vi "WaterValve.vi"(9 "Max pulses":u32=1, 11 "STOP":bool) -> (1 "Error":bool, 3 "Number pulses":u32)   [LabVIEW 2021]
uses:
  <vilib>/DAQmx/write.llb/DAQmx Write (Digital Bool 1Line 1Point).vi
  GlobalSTATE.vi
  <vilib>/DAQmx/create/channels.llb/DAQmx Create Channel (DO-Digital Output).vi
  Global_BeamBreaks.vi
  <vilib>/DAQmx/miscellaneous.llb/DAQmx Fill In Error Info.vi
panel:
  in  "Active":bool=TRUE
  in  "Min IPI":u32=500
  in  "Open time":u32=50
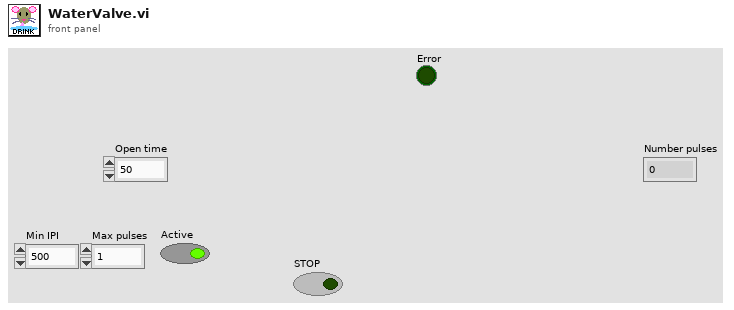
[diagram p1: front panel]
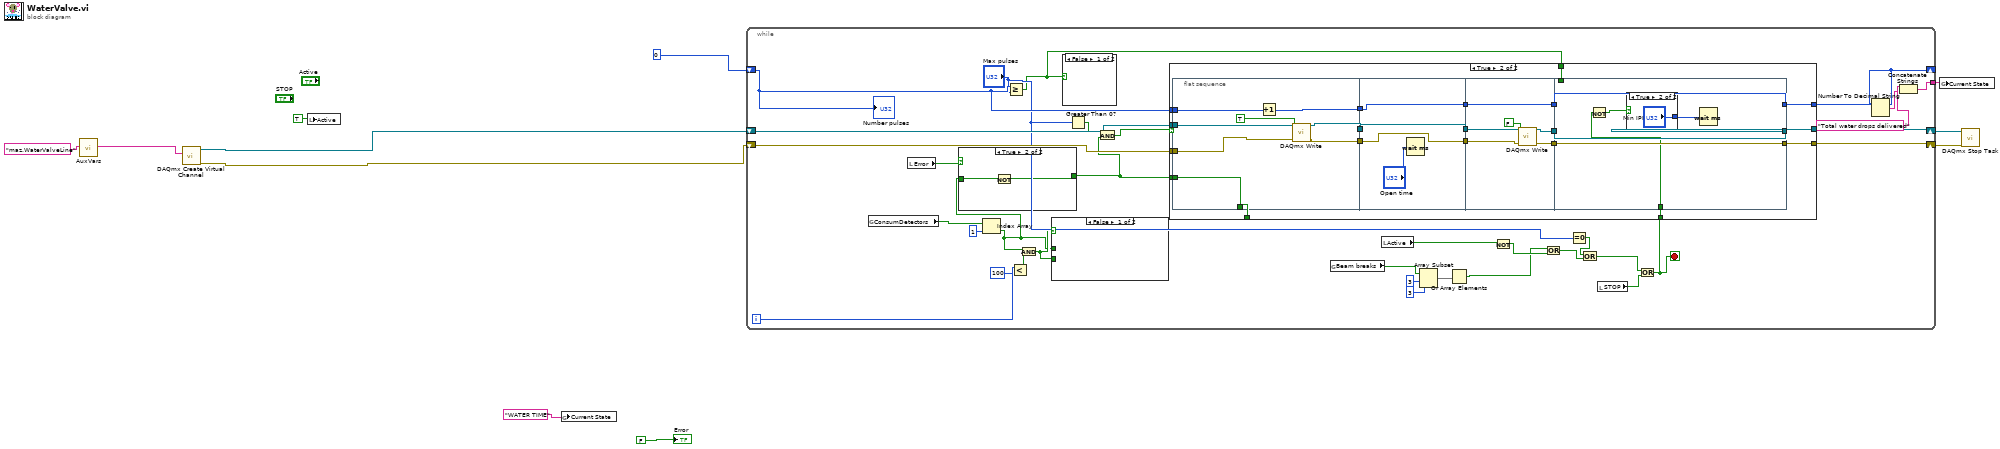
[diagram p0: block diagram]
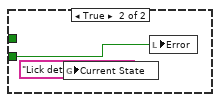
[diagram p3: hidden frame]
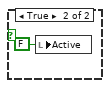
[diagram p4: hidden frame]
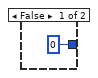
[diagram p6: hidden frame]
diagram:
  n1 = call "AuxVars.vi"("key"="maz.WaterValveLine") -> ("value"=w7:string)  [unwired: 9 in, 1 out]
  n2 = call-poly <vilib>:"DAQmx Create Virtual Channel.vi"("lines"=w7) -> ("task out"=w9:refnum<k21>, "error out"=w8:errorcluster)  [unwired: 13 in]
  n3 = local write "Active"(TRUE ("Active")) -> ()
  n4 = global write "GlobalSTATE.vi" "Current State"("WATER TIME" ("Current State")) -> ()
  n5 = while {
    shift-right: [w43] -> w4
    shift-left: w9 -> [w45]
    shift-right: [w42] -> w3
    shift-left: w8 -> [w44]
    shift-right: [w33] -> _
    shift-left: 0 -> [w41]
    tunnel: [w32] -> w2
    i -> [w17]
    stop <- w23 stop-if-true
    n6 = global read "Global_BeamBreaks.vi" "ConsumDetectors"() -> (w20:bool[])
    n7 = local read "Error"() -> (w14:bool)
    n8 = Index Array(array=w20, index=1) -> (element=w13:bool)
    n9 = case shown="True" w14 {
      tunnel: w13 -> [w46 w48]
      tunnel: [w46 w47] -> w12
      frame False {
      }
      frame True {
        n10 = Not(x=w48) -> (.not. x?=w47:bool)
      }
    }
    n11 = Greater Or Equal?(x=w41, y="Max pulses") -> (x >= y?=w31:bool)
    n12 = Less?(x=w17, y=100) -> (x < y?=w18:bool)
    n13 = And(x=w13, y=w18) -> (x .and. y?=w15:bool)
    n14 = case shown="False" w15 {
      tunnel: w13 -> [_ _]
      tunnel: w15 -> [_ w49]
      frame False {
      }
      frame True {
        n15 = global write "GlobalSTATE.vi" "Current State"("Lick detector ERROR") -> ()
        n16 = local write "Error"(w49) -> ()
      }
    }
    n17 = case shown="False" w31 {
      frame False {
      }
      frame True {
        n18 = local write "Active"(FALSE ("Active")) -> ()
      }
    }
    n19 = Greater Than 0?(x="Max pulses") -> (x > 0?=w38:bool)
    n20 = And(x=w38, y=w12) -> (x .and. y?=w37:bool)
    n21 = global read "Global_BeamBreaks.vi" "Beam breaks"() -> (w26:bool[])
    n22 = local read "Active"() -> (w40:bool)
    n23 = Array Subset(array=w26, index=3, length=3) -> (w25:bool[])
    n24 = Or Array Elements(Boolean array=w25) -> (logical OR=w24:bool)
    n25 = Not(x=w40) -> (.not. x?=w39:bool)
    n26 = Or(x=w24, y=w39) -> (x .or. y?=w36:bool)
    n27 = Equal To 0?(x="Max pulses") -> (x = 0?=w35:bool)
    n28 = Or(x=w35, y=w36) -> (x .or. y?=w29:bool)
    n29 = local read "STOP"() -> (w30:bool)
    n30 = Or(x=w29, y=w30) -> (x .or. y?=w23:bool)
    n31 = case shown="True" w37 {
      tunnel: w45 -> [w55 w70]
      tunnel: w44 -> [w54 w69]
      tunnel: [w55 w68] -> w43
      tunnel: [w54 w67] -> w42
      tunnel: w12 -> [w53 w66]
      tunnel: [w53 w65] -> _
      tunnel: w41 -> [w52 w61]
      tunnel: [w52 w58] -> w33
      tunnel: w31 -> [_ w57]
      tunnel: w23 -> [_ w56]
      frame False {
      }
      frame True {
        n32 = flat-sequence {
          tunnel: w70 -> [w82]
          tunnel: w69 -> [w81]
          tunnel: [w79] -> w74
          tunnel: [w78] -> w73
          tunnel: w66 -> [w77]
          tunnel: [w77] -> w65
          tunnel: [w75] -> w62
          tunnel: w61 -> [w76]
          tunnel: [w85] -> w72
          tunnel: w74 -> [w85]
          tunnel: [w84] -> w71
          tunnel: w73 -> [w84]
          tunnel: w62 -> [w83]
          tunnel: [w83] -> w59
          tunnel: w72 -> [w91]
          tunnel: w71 -> [w90]
          tunnel: [w89] -> w64
          tunnel: [w88] -> w63
          tunnel: [w87] -> w60
          tunnel: w59 -> [w87]
          tunnel: [w97] -> w67
          tunnel: [w98] -> w68
          tunnel: w64 -> [w98]
          tunnel: w63 -> [w97]
          tunnel: w60 -> [w95]
          tunnel: [w95] -> w58
          tunnel: w57 -> [_]
          tunnel: w56 -> [w93]
          frame #0 {
            n33 = Increment(x=w76) -> (x+1=w75:i32)
            n34 = call-poly <vilib>:"DAQmx Write.vi"("task/channels in"=w82, "data"=TRUE, "error in"=w81) -> ("task out"=w79:refnum<k21>, "error out"=w78:errorcluster)  [unwired: 10 in, 1 out]
          }
          frame #1 {
            n35 = Wait (ms)(milliseconds to wait="Open time") -> ()  [unwired: 1 out]
          }
          frame #2 {
            n36 = call-poly <vilib>:"DAQmx Write.vi"("task/channels in"=w91, "data"=FALSE, "error in"=w90) -> ("task out"=w89:refnum<k21>, "error out"=w88:errorcluster)  [unwired: 10 in, 1 out]
          }
          frame #3 {
            n37 = Not(x=w93) -> (.not. x?=w94:bool)
            n38 = case shown="True" w94 {
              tunnel: [u32 0 ("Min IPI") "Min IPI"] -> w96
              frame False {
              }
              frame True {
              }
            }
            n39 = Wait (ms)(milliseconds to wait=w96) -> ()  [unwired: 1 out]
          }
        }
      }
    }
    n40 = Number To Decimal String(number=w33) -> (decimal integer string=w21:string)  [unwired: 1 in]
    n41 = Concatenate Strings("Total water drops delivered" ("string"), w21) -> (w32:string)
    "Number pulses" <- w41
  }
  n42 = global write "GlobalSTATE.vi" "Current State"(w2) -> ()
  n43 = call <vilib>:"DAQmx Stop Task.vi"("task/channels in"=w4, "error in"=w3) -> ()  [unwired: 12 in, 2 out]
  "Error" <- FALSE ("Error")
